vi "Move Window.vi"(8 "error in (no error)":errorcluster, 10 "window position":cluster{"Left":i16, "Top":i16}, 11 "VI Ref":refnum<vi>) -> (0 "error out":errorcluster)   [LabVIEW 2017, in "DSF Core.lvlib"]
uses:
  DSF Core.lvlib
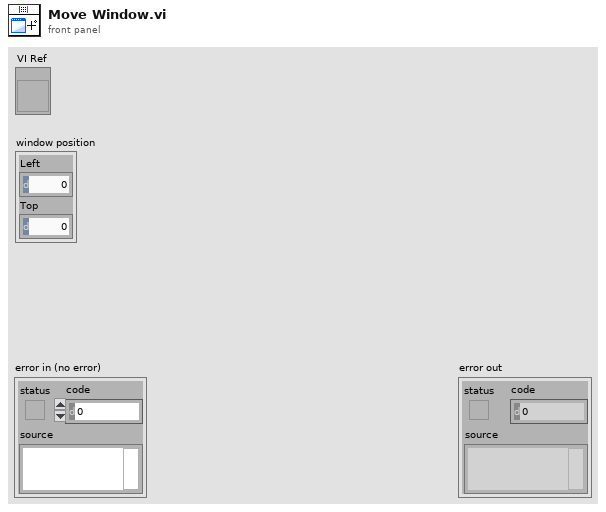
[diagram p1: front panel]
types:
  T1 = typedef "LVRectTypeDef.ctl" = cluster{"Left":i16, "Top":i16, "Right":i16, "Bottom":i16}
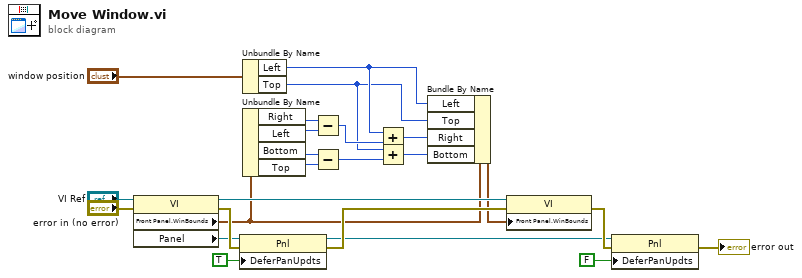
[diagram p0: block diagram]
diagram:
  n1 = property class="VI"(reference="VI Ref", error in="error in (no error)") -> (reference out=w3:refnum<vi>, error out=w12:errorcluster, "Front Panel.WinBounds"=w1:T1, "Panel"=w4:refnum<vi>)
  n2 = property class="Pnl"(reference=w4, error in=w12, "DeferPanUpdts"=TRUE ("Defer Panel Updates")) -> (reference out=w9:refnum<vi>, error out=w24:errorcluster)
  n3 = Unbundle By Name("window position") -> ("Left"=w19:i16, "Top"=w16:i16)
  n4 = Unbundle By Name(w1) -> ("Right"=w23:i16, "Left"=w22:i16, "Bottom"=w21:i16, "Top"=w20:i16)
  n5 = Subtract(x=w23, y=w22) -> (x-y=w17:i16)
  n6 = Subtract(x=w21, y=w20) -> (x-y=w14:i16)
  n7 = Add(x=w19, y=w17) -> (x+y=w18:i16)
  n8 = Add(x=w16, y=w14) -> (x+y=w15:i16)
  n9 = Bundle By Name(cluster=w1, "Left"=w19, "Top"=w16, "Right"=w18, "Bottom"=w15) -> (w2:T1)
  n10 = property class="VI"(reference=w3, error in=w24, "Front Panel.WinBounds"=w2) -> (error out=w10:errorcluster)  [unwired: 1 out]
  n11 = property class="Pnl"(reference=w9, error in=w10, "DeferPanUpdts"=FALSE ("Defer Panel Updates")) -> (error out=→"error out":errorcluster)  [unwired: 1 out]
